vi "AM Update.vi"(8 "error in (no error)":errorcluster, 10 "Message Queues in":T1, 11 "Data Cluster":T2) -> (0 "error out":errorcluster, 3 "Data Cluster out":T2)   [LabVIEW 2020, in "Motion.lvlib"]
uses:
  Motion.lvlib
  AM Configuration.ctl
  support/Message Queue/Message Cluster.ctl
  support/Message Queue/Message Queue.lvlib
  support/Message Queue/All Message Queues.ctl
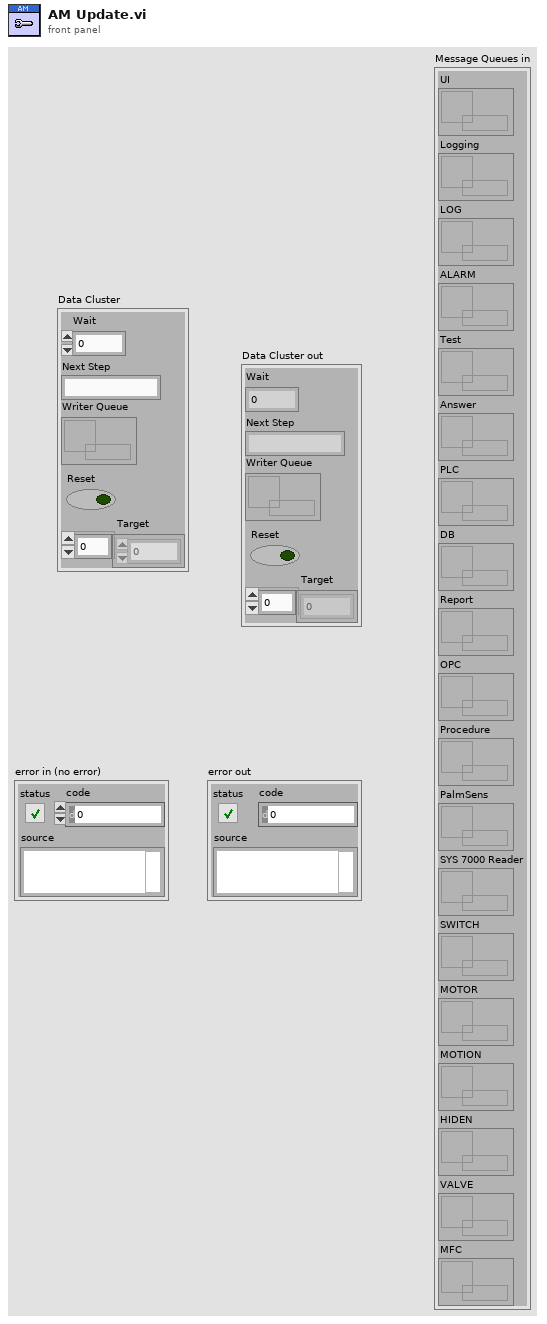
[diagram p1: front panel]
types:
  T1 = typedef "Message Queue.lvlib/All Message Queues.ctl" = cluster{"UI":refnum<queue>, "Logging":refnum<queue>, "LOG":refnum<queue>, "ALARM":refnum<queue>, "Test":refnum<queue>, "Answer":refnum<queue>, "PLC":refnum<queue>, "DB":refnum<queue>, "Report":refnum<queue>, "OPC":refnum<queue>, "Procedure":refnum<queue>, "PalmSens":refnum<queue>, "SYS 7000 Reader":refnum<queue>, "SWITCH":refnum<queue>, "MOTOR":refnum<queue>, "MOTION":refnum<queue>, "HIDEN":refnum<queue>, "VALVE":refnum<queue>, "MFC":refnum<queue>}
  T2 = typedef "Motion.lvlib/AM Configuration.ctl" = cluster{"Wait":dbl, "Next Step":string, "Writer Queue":refnum<queue>, "Reset":bool, "Target":dbl[]}
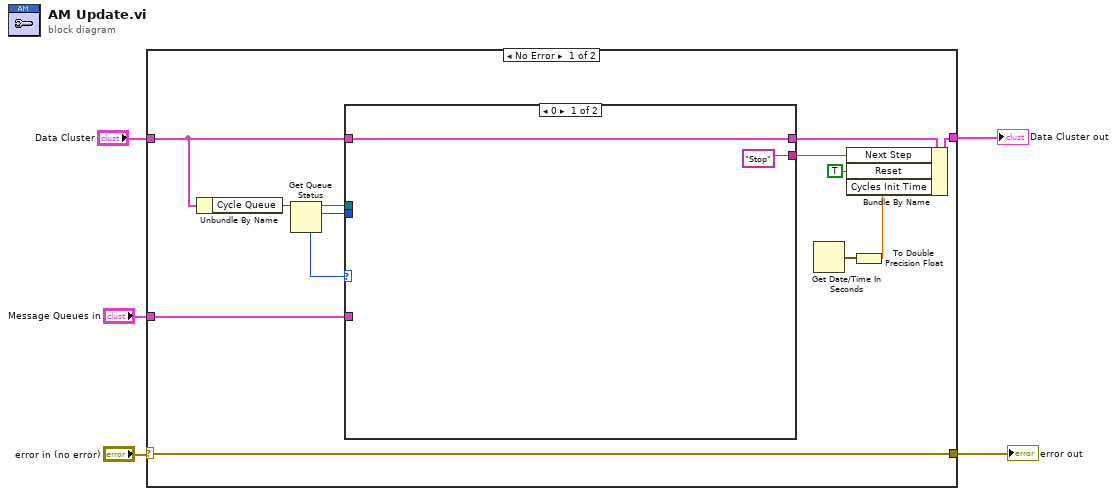
[diagram p0: block diagram]
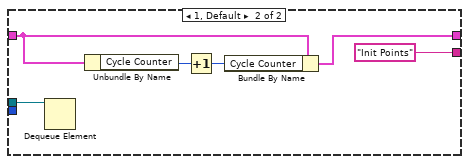
[diagram p2: hidden frame]
diagram:
  n1 = case shown="No Error" "error in (no error)" {
    selector: "error in (no error)" -> [w18 w27]
    tunnel: [w13 w28] -> w4
    tunnel: "Data Cluster" -> [w15 w28]
    tunnel: [w18 w27] -> w3
    tunnel: "Message Queues in" -> [w9 _]
    frame No Error {
      n2 = Unbundle By Name(w15) -> ("Cycle Queue"=w17:refnum<queue>)
      n3 = Get Queue Status(queue=w17) -> (queue out=w16:refnum<queue>, # pending remove=w8:i32, # elements in queue=w10:i32)  [unwired: 2 in, 5 out]
      n4 = case shown="0" w10 {
        tunnel: w16 -> [_ w26]
        tunnel: [w19 w22] -> w14
        tunnel: w15 -> [w19 w21]
        tunnel: ["Stop" "Init Points"] -> w12
        tunnel: w9 -> [_ _]
        tunnel: w8 -> [_ _]
        frame 0 {
        }
        frame 1, Default {
          n5 = Dequeue Element(queue=w26) -> ()  [unwired: 2 in, 4 out]
          n6 = Unbundle By Name(w21) -> ("Cycle Counter"=w24:i32)
          n7 = Increment(x=w24) -> (x+1=w23:i32)
          n8 = Bundle By Name(cluster=w21, "Cycle Counter"=w23) -> (w22:T2)
        }
      }
      n9 = Get Date/Time In Seconds() -> (seconds since 1Jan1904=w7:timestamp)
      n10 = To Double Precision Float(number=w7) -> (double precision float=w6:dbl)
      n11 = Bundle By Name(cluster=w14, "Next Step"=w12, "Reset"=TRUE, "Cycles Init Time"=w6) -> (w13:T2)
    }
    frame Error {
    }
  }
  "error out" <- w3
  "Data Cluster out" <- w4
